vi "ASTZ - AVL Sesam.vi"(10 "Selektor":string) -> (2 "Verknüpfter String":string)   [LabVIEW 2020, in "AK-Schnittstelle.lvlib"]
uses:
  AK-Schnittstelle.lvlib
  Funktionstasten/Funktionstasten-Aktion.ctl
  Aktionen Gespeicherte Werte.ctl
  Funktionstasten/Funktionstasten.lvlib
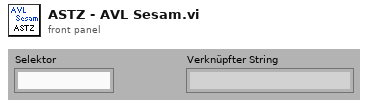
[diagram p1: front panel]
types:
  T1 = typedef "AK-Schnittstelle.lvlib/Aktionen Gespeicherte Werte.ctl" = enum16{"lesen", "laden", "speichern", "Seriell", "TCP", "Diverse", "AKTIV", "AK-Namen"}
  T2 = typedef "Funktionstasten.lvlib/Funktionstasten-Aktion.ctl" = enum16{"Initialisieren", "Zustand setzen", "Taste gedrückt", "Fehler speichern", "Lesen", "Manuell", "Remote", "Bitparallel", "Samplepoint", "Zeit Prüfen", "reset Umschalten"}
  T3 = typedef "Funktionstasten.lvlib/Zustaende.ctl" = enum16{"Standby", "Pause", "Eco", "Messen", "Kalibrieren", "Spülen Filter", "Spülen Leitung", "Umgebungsluft", "0-Gas", "Cal-Gas", "CG zu PNS", "-------------", "Init 1", "Init 2", "Init 3", "Init 4", "Messen vorbereiten", "Messen durchführen", "Exit"}
  T4 = typedef "Funktionstasten.lvlib/Betriebsart.ctl" = enum16{"Manuell", "Remote", "Bitparallel"}
  T5 = typedef "AK-Schnittstelle.lvlib/Diverse gespeicherte Werte.ctl" = cluster{"Kalibriergaseingang":i16, "SamplePoint":i16, "CalGas zu PNS":i16, "Gas-Reihenfolge":i16[], "Zeit 0-Gas":sgl, "Zeit CalGas":sgl, "AK Befehlssatz":T6}
  T6 = typedef "AK-Schnittstelle.lvlib/AK Befehlssatz.ctl" = enum16{"MEXA", "IAG v1.4", "AVL (Puma)", "PEUS"}
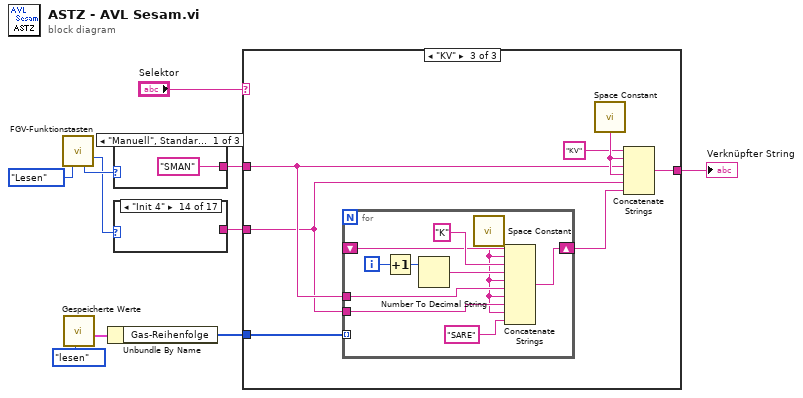
[diagram p0: block diagram]
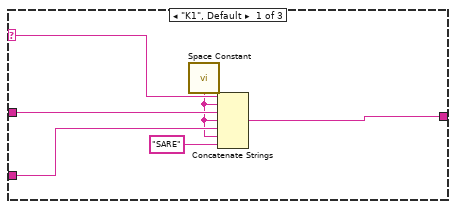
[diagram p2: hidden frame]
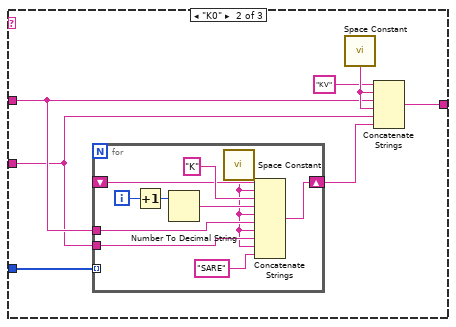
[diagram p3: hidden frame]
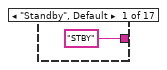
[diagram p4: hidden frame]
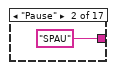
[diagram p5: hidden frame]
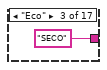
[diagram p6: hidden frame]
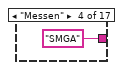
[diagram p7: hidden frame]
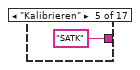
[diagram p8: hidden frame]
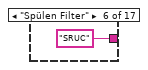
[diagram p9: hidden frame]
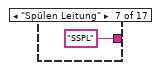
[diagram p10: hidden frame]
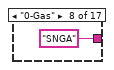
[diagram p11: hidden frame]
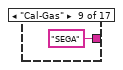
[diagram p12: hidden frame]
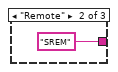
[diagram p20: hidden frame]
diagram:
  n1 = call "FGV-Funktionstasten.vi"("Aktion"=Funktionstasten-Aktion."Lesen") -> ("ausgewählte Funktion"=w8:T3, "Betriebsart"=w9:T4)  [unwired: 7 in, 6 out]
  n2 = call "Gespeicherte Werte.vi"("Aktionen"=Aktionen_Gespeicherte_Werte."lesen") -> ("Diverse Werte"=w5:T5)  [unwired: 6 in, 4 out]
  n3 = Unbundle By Name(w5) -> ("Gas-Reihenfolge"=w1:i16[])
  n4 = case shown="\"Manuell\", Standard" w9 {
    tunnel: ["SMAN" ("String") "SREM" ("String") "SBIT" ("String")] -> w4
    frame "Manuell", Default {
    }
    frame "Remote" {
    }
    frame "Bitparallel" {
    }
  }
  n5 = case shown="\"Init 4\"" w8 {
    tunnel: ["STBY" ("String") "SPAU" ("String") "SECO" ("String") "SMGA" ("String") "SATK" ("String") "SRUC" ("String") "SSPL" ("String") "SNGA" ("String") "SEGA" ("String") _ _ _ _ _ _ _ _] -> w3
    frame "Standby", Default {
    }
    frame "Pause" {
    }
    frame "Eco" {
    }
    frame "Messen" {
    }
    frame "Kalibrieren" {
    }
    frame "Spülen Filter" {
    }
    frame "Spülen Leitung" {
    }
    frame "0-Gas" {
    }
    frame "Cal-Gas" {
    }
    frame "-------------" {
    }
    frame "Init 1" {
    }
    frame "Init 2" {
    }
    frame "Init 3" {
    }
    frame "Init 4" {
    }
    frame "Messen vorbereiten" {
    }
    frame "Messen durchführen" {
    }
    frame "Exit" {
    }
  }
  n6 = case shown="\"KV\"" "Selektor" {
    selector: "Selektor" -> [w28 _ _]
    tunnel: [w23 w29 w46] -> w2
    tunnel: w4 -> [w27 w32 w49]
    tunnel: w3 -> [w26 w31 w48]
    tunnel: w1 -> [_ w33 w47]
    frame "K1", Default {
      n7 = call <vilib>:"Space Constant.vi"() -> ("String"=w25:string)
      n8 = Concatenate Strings(w28, w25, w27, w25, w26, w25, "SARE" ("String")) -> (w23:string)
    }
    frame "K0" {
      n9 = for {
        tunnel: w33 -> [_] mode=indexing
        shift-right: [w41] -> w30
        shift-left: _ -> [w42]
        tunnel: w32 -> [w39]
        tunnel: w31 -> [w38]
        i -> [w44]
        n10 = Increment(x=w44) -> (x+1=w45:i32)
        n11 = Number To Decimal String(number=w45) -> (decimal integer string=w40:string)  [unwired: 1 in]
        n12 = call <vilib>:"Space Constant.vi"() -> ("String"=w37:string)
        n13 = Concatenate Strings(w42, w37, "K" ("String"), w40, w37, w39, w37, w38, w37, "SARE" ("String")) -> (w41:string)
      }
      n14 = call <vilib>:"Space Constant.vi"() -> ("String"=w35:string)
      n15 = Concatenate Strings("KV" ("String"), w35, w32, w35, w31, w30) -> (w29:string)
    }
    frame "KV" {
      n16 = for {
        tunnel: w47 -> [_] mode=indexing
        shift-right: [w58] -> w50
        shift-left: _ -> [w59]
        tunnel: w49 -> [w56]
        tunnel: w48 -> [w55]
        i -> [w61]
        n17 = Increment(x=w61) -> (x+1=w62:i32)
        n18 = Number To Decimal String(number=w62) -> (decimal integer string=w57:string)  [unwired: 1 in]
        n19 = call <vilib>:"Space Constant.vi"() -> ("String"=w54:string)
        n20 = Concatenate Strings(w59, w54, "K" ("String"), w57, w54, w56, w54, w55, w54, "SARE" ("String")) -> (w58:string)
      }
      n21 = call <vilib>:"Space Constant.vi"() -> ("String"=w52:string)
      n22 = Concatenate Strings("KV" ("String"), w52, w49, w52, w48, w50) -> (w46:string)
    }
  }
  "Verknüpfter String" <- w2
